vi "3D_scanner.vi"(0 "pixel_dwell_ms":dbl=0.1 caption="Dwell time:", 1 "pos-start_x":dbl, 2 "pos-start_y":dbl, 3 "enable":refnum<vi>, 5 "frame_size_x_px":i32=50, 7 "image_size_x_um":dbl=6.0, 9 "pos_start":enum32{"bottom-left", "center"}(ring), 10 "z-stack_enable":bool, 11 "scan_direction":enum32{"0", "1"}(radio)=enum."1" caption="Scan direction:", 12 "IntensityGraph in":refnum<vi>, 13 "z_start":dbl format="%0.2f", 14 "z_end":dbl=1.0 format="%0.2f", 15 "z_q_slices":i32=128) -> (6 "image_out":dbl[][][](array[numeric]))   [LabVIEW 2014]
uses:
  <vilib>/Analysis/1siggen.llb/Ramp Pattern by Samples.vi
  <vilib>/Analysis/NI_AALBase.lvlib
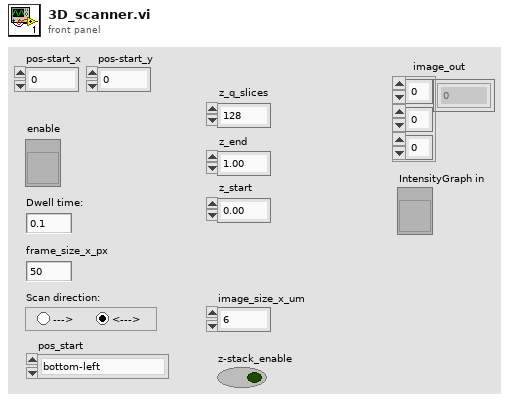
[diagram p1: front panel]
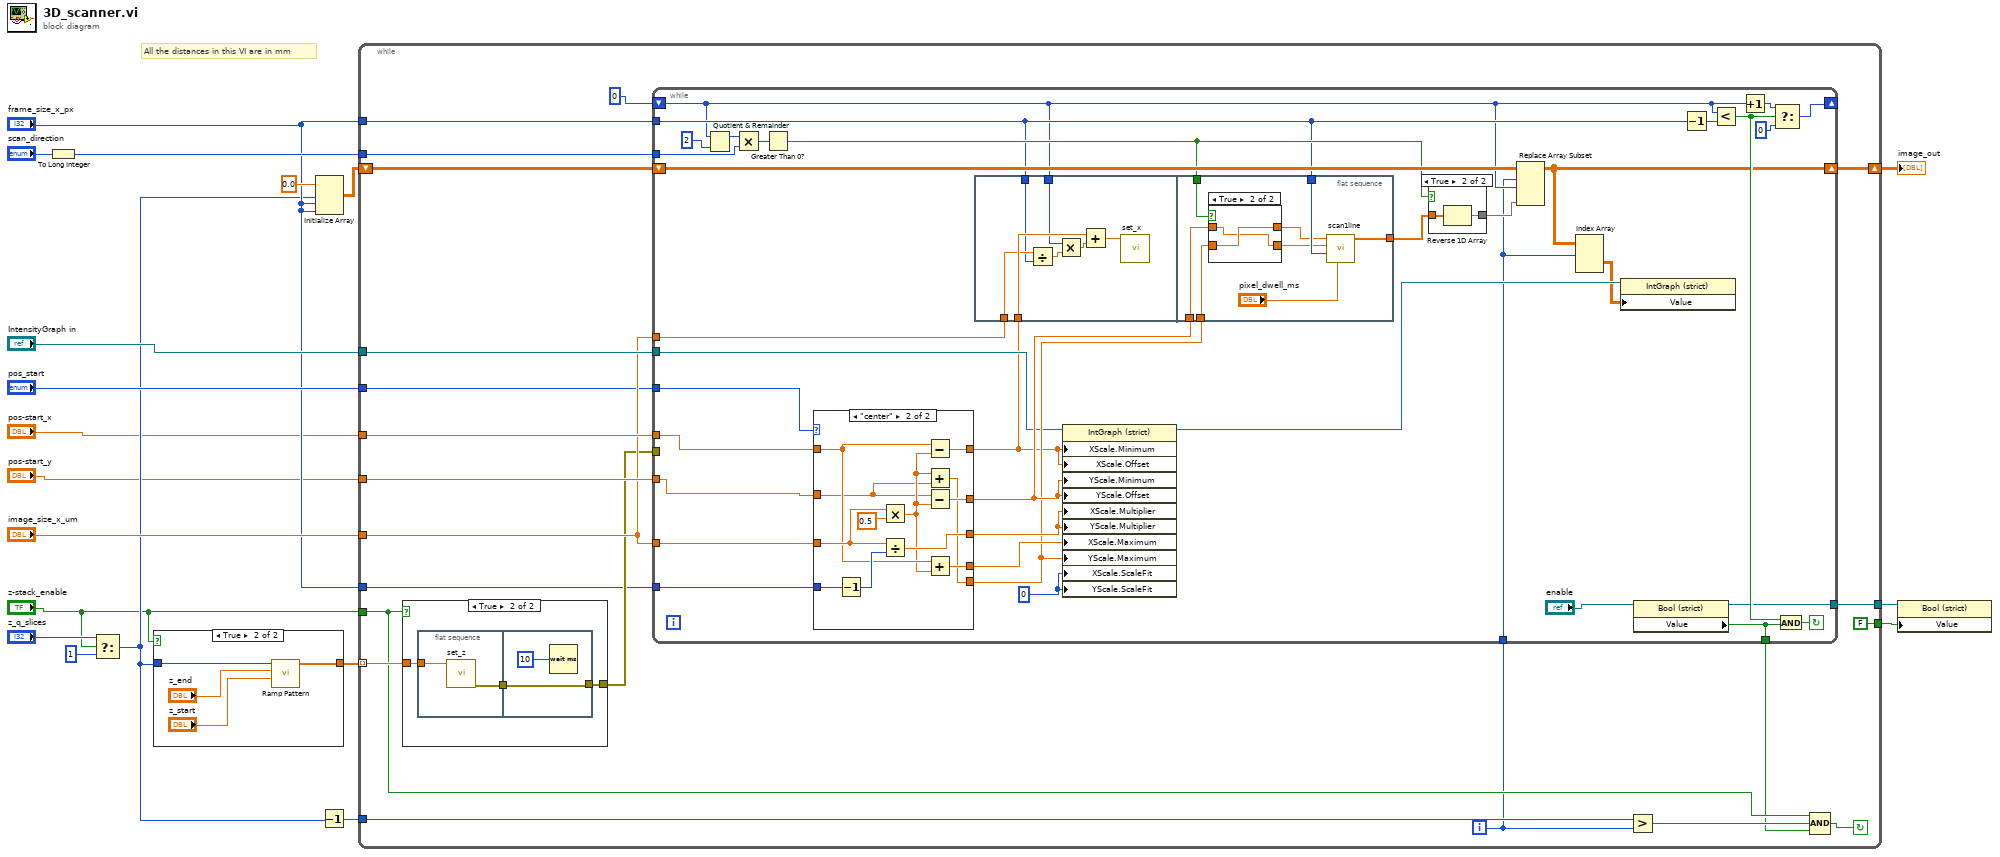
[diagram p0: block diagram]
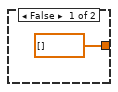
[diagram p2: hidden frame]
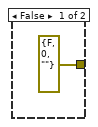
[diagram p3: hidden frame]
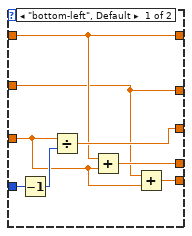
[diagram p6: hidden frame]
diagram:
  # "All the distances in this VI are in mm"
  n1 = To Long Integer(number="scan_direction") -> (32bit integer=w17:i32)
  n2 = Select(t="z_q_slices", s="z-stack_enable", f=1) -> (s? t:f=w4:i32)
  n3 = case shown="True" "z-stack_enable" {
    tunnel: [dbl[] [] ("Ramp Pattern") w22] -> w14
    tunnel: w4 -> [_ w21]
    frame False {
    }
    frame True {
      n4 = call-poly <vilib>:"Ramp Pattern.vi"("start"="z_start", "end"="z_end", "samples"=w21) -> ("Ramp Pattern"=w22:dbl[])  [unwired: 7 in, 1 out]
    }
  }
  n5 = Initialize Array(0.0 ("element"), w4, "frame_size_x_px", "frame_size_x_px") -> (w9:dbl[][][])
  n6 = Decrement(x=w4) -> (x-1=w12:i32)
  n7 = while {
    tunnel: "pos-start_x" -> [w44]
    tunnel: "pos-start_y" -> [w43]
    tunnel: "IntensityGraph in" -> [w42]
    tunnel: w17 -> [w41]
    tunnel: "frame_size_x_px" -> [w31]
    tunnel: "image_size_x_um" -> [w40]
    tunnel: "pos_start" -> [w39]
    tunnel: w12 -> [w32]
    tunnel: w14 -> [w37] mode=indexing
    tunnel: "z-stack_enable" -> [w34]
    tunnel: "frame_size_x_px" -> [w30]
    shift-right: [w29] -> w11
    shift-left: w9 -> [w27]
    tunnel: [w26] -> w7
    tunnel: [FALSE ("Value")] -> w6
    i -> [w28]
    stop <- w36 continue-if-true
    n8 = case shown="True" w34 {
      tunnel: [errorcluster {"status"=FALSE, "code"=0, "source"=""} ("error out") w48] -> w38
      tunnel: w37 -> [_ w47]
      frame False {
      }
      frame True {
        n9 = flat-sequence {
          tunnel: w47 -> [w50]
          tunnel: [w51] -> w49
          tunnel: [w52] -> w48
          tunnel: w49 -> [w52]
          frame #0 {
            n10 = call "set_z.vi"("z_value_um"=w50) -> ("error out"=w51:errorcluster)  [unwired: 10 in]
          }
          frame #1 {
            n11 = Wait (ms)(milliseconds to wait=u32 10) -> ()  [unwired: 1 out]
          }
        }
      }
    }
    n12 = while {
      shift-right: [w59] -> w29
      shift-left: w27 -> [w89]
      shift-right: [w88] -> _
      shift-left: 0 -> [w60]
      tunnel: w31 -> [w71]
      tunnel: w44 -> [w55]
      tunnel: w43 -> [w54]
      tunnel: w40 -> [w67]
      tunnel: w42 -> [w74]
      tunnel: w41 -> [w73]
      tunnel: w30 -> [w69]
      tunnel: w40 -> [w68]
      tunnel: w39 -> [w66]
      tunnel: w38 -> [_]
      tunnel: [w62] -> w33
      tunnel: w28 -> [w58]
      tunnel: [w56] -> w26
      stop <- w63 continue-if-true
      w65 = u8 0 ("X Scale.Scale Fit")
      n13 = Quotient & Remainder(x=w60, y=2) -> (x-y*floor(x/y)=w81:i32)  [unwired: 1 out]
      n14 = Multiply(x=w81, y=w73) -> (x*y=w80:i32)
      n15 = Greater Than 0?(x=w80) -> (x > 0?=w77:bool)
      n16 = case shown="\"center\"" w66 {
        tunnel: w55 -> [w116 w125]
        tunnel: w54 -> [w113 w122]
        tunnel: w67 -> [w114 w129]
        tunnel: [w116 w126] -> w72
        tunnel: [w113 w127] -> w76
        tunnel: [w118 w130] -> w84
        tunnel: [w117 w124] -> w83
        tunnel: [w115 w121] -> w75
        tunnel: w69 -> [w112 w120]
        frame "bottom-left", Default {
          n17 = Decrement(x=w112) -> (x-1=w119:i32)
          n18 = Divide(x=w114, y=w119) -> (x/y=w118:dbl)
          n19 = Add(x=w116, y=w114) -> (x+y=w117:dbl)
          n20 = Add(x=w113, y=w114) -> (x+y=w115:dbl)
        }
        frame "center" {
          n21 = Decrement(x=w120) -> (x-1=w131:i32)
          n22 = Multiply(x=w129, y=0.5) -> (x*y=w123:dbl)
          n23 = Divide(x=w129, y=w131) -> (x/y=w130:dbl)
          n24 = Subtract(x=w125, y=w123) -> (x-y=w126:dbl)
          n25 = Add(x=w123, y=w122) -> (x+y=w121:dbl)
          n26 = Subtract(x=w122, y=w123) -> (x-y=w127:dbl)
          n27 = Add(x=w125, y=w123) -> (x+y=w124:dbl)
        }
      }
      n28 = flat-sequence {
        tunnel: w72 -> [w96]
        tunnel: w60 -> [w94]
        tunnel: w68 -> [w92]
        tunnel: w71 -> [w91]
        tunnel: [w103] -> w79
        tunnel: w71 -> [w102]
        tunnel: w77 -> [w99]
        tunnel: w76 -> [w98]
        tunnel: w75 -> [w97]
        frame #0 {
          n29 = Divide(x=w92, y=w91) -> (x/y=w93:dbl)
          n30 = Multiply(x=w94, y=w93) -> (x*y=w95:dbl)
          n31 = Add(x=w96, y=w95) -> (x+y=w90:dbl)
          n32 = call "set_x.vi"("x_value_um"=w90) -> ()  [unwired: 10 in, 1 out]
        }
        frame #1 {
          n33 = case shown="True" w99 {
            tunnel: [w105 w108] -> w101
            tunnel: [w106 w107] -> w100
            tunnel: w97 -> [w106 w108]
            tunnel: w98 -> [w105 w107]
            frame False {
            }
            frame True {
            }
          }
          n34 = call "scan1line.vi"("dwell_time_ms"="pixel_dwell_ms", "q_pixels"=w102, "y_end"=w100, "y_start"=w101) -> ("histogram plot"=w103:dbl[])  [unwired: 6 in, 1 out]
        }
      }
      n35 = property on="Property Node" class="IntGraph (strict)"(reference=w74, "XScale.Minimum"=w72, "XScale.Offset"=w72, "YScale.Minimum"=w76, "YScale.Offset"=w76, "XScale.Multiplier"=w84, "YScale.Multiplier"=w84, "XScale.Maximum"=w83, "YScale.Maximum"=w75, "XScale.ScaleFit"=w65, "YScale.ScaleFit"=w65) -> (reference out=w70:refnum<vi>)  [unwired: 1 in, 1 out]
      n36 = case shown="True" w77 {
        tunnel: w79 -> [w109 w111]
        tunnel: [w109 w110] -> w78
        frame False {
        }
        frame True {
          n37 = Reverse 1D Array(array=w111) -> (reversed array=w110:dbl[])
        }
      }
      n38 = Replace Array Subset(array=w89, new element=w78, index (dim 0)=w58, index (dim 1)=w60) -> (w59:dbl[][][])  [unwired: 1 in]
      n39 = Index Array(array=w59, index (dim 0)=w58) -> (element=w57:dbl[][])  [unwired: 2 in]
      n40 = property on="Property Node" class="IntGraph (strict)"(reference=w70, "Value"=w57) -> ()  [unwired: 1 in, 2 out]
      n41 = property class="Bool (strict)"(reference="enable") -> (reference out=w56:refnum<vi>, "Value"=w62:bool)  [unwired: 1 in, 1 out]
      n42 = Decrement(x=w71) -> (x-1=w85:i32)
      n43 = Less?(x=w60, y=w85) -> (x < y?=w64:bool)
      n44 = Increment(x=w60) -> (x+1=w87:i32)
      n45 = Select(t=w87, s=w64, f=0) -> (s? t:f=w88:i32)
      n46 = And(x=w64, y=w62) -> (x .and. y?=w63:bool)
    }
    n47 = Greater?(x=w32, y=w28) -> (0:w35:bool)
    n48 = Compound Arithmetic op=AND(w34, w35, w33) -> (w36:bool)
  }
  "image_out" <- w11
  n49 = property class="Bool (strict)"(reference=w7, "Value"=w6) -> ()  [unwired: 1 in, 2 out]
